vi "test.vi"() -> ()   [LabVIEW 2022 SP3]
panel:
  in  "stop":bool
  in  "volume":i32
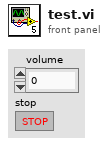
[diagram p1: front panel]
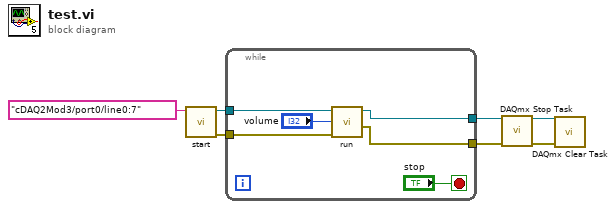
[diagram p0: block diagram]
diagram:
  n1 = call "start.vi"("lines"=tag "cDAQ2Mod3/port0/line0:7") -> ("error out"=w5:errorcluster, "Refnum out"=w6:refnum<k21>)  [unwired: 9 in]
  n2 = while {
    tunnel: w6 -> [w10]
    tunnel: w5 -> [w11]
    tunnel: [w9] -> w2
    tunnel: [w8] -> w1
    stop <- "stop" stop-if-true
    n3 = call "run.vi"("error in (no error)"=w11, "volume"="volume", "Refnum in"=w10) -> ("error out"=w8:errorcluster, "Refnum out"=w9:refnum<k21>)  [unwired: 7 in]
  }
  n4 = call <vilib>:"DAQmx Stop Task.vi"("task/channels in"=w2, "error in"=w1) -> ("task out"=w4:refnum<k21>, "error out"=w3:errorcluster)  [unwired: 12 in]
  n5 = call <vilib>:"DAQmx Clear Task.vi"("task in"=w4, "error in"=w3) -> ()  [unwired: 13 in, 1 out]
